vi "Header_Info_Str.vi"(8 "error in (no error)":errorcluster, 10 "Functions":i32, 11 "DefaultDev in":refnum<class "BaseDevice.lvclass">) -> (0 "error out":errorcluster, 1 "HdrInfoStr":string, 2 "InstrumentName":string, 3 "DefaultDev out":refnum<class "BaseDevice.lvclass">)   [LabVIEW 2019, in "BaseDevice.lvclass"]
uses:
  BaseDevice.lvclass
  BaseDevice.lvclass/BaseDevice.ctl
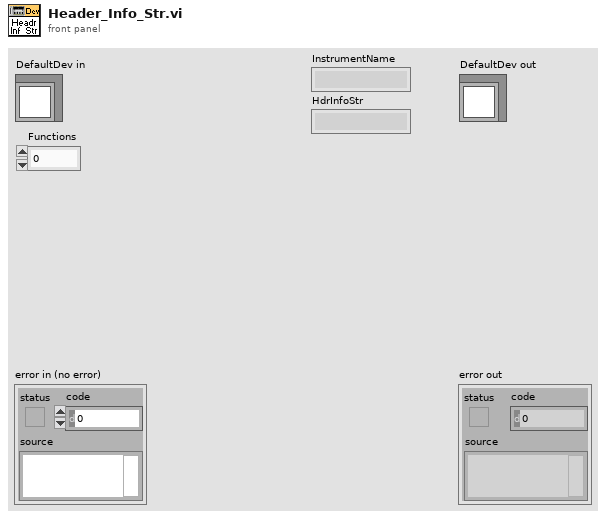
[diagram p1: front panel]
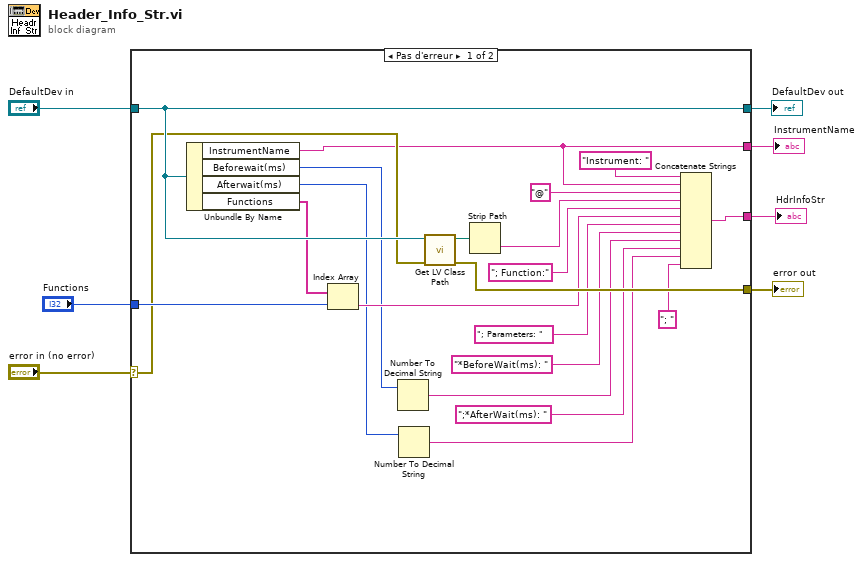
[diagram p0: block diagram]
diagram:
  n1 = case shown="Pas d'erreur" "error in (no error)" {
    selector: "error in (no error)" -> [w13 w30]
    tunnel: [w24 w30] -> w6
    tunnel: [w18 w29] -> w4
    tunnel: "DefaultDev in" -> [w18 w29]
    tunnel: [w12 _] -> w3
    tunnel: [w15 _] -> w2
    tunnel: "Functions" -> [w14 _]
    frame No Error {
      n2 = Unbundle By Name(w18) -> ("InstrumentName"=w12:string, "Beforewait(ms)"=w11:u32, "Afterwait(ms)"=w10:u32, "Functions"=w9:string[])
      n3 = Index Array(array=w9, index=w14) -> (element=w17:string)
      n4 = Number To Decimal String(number=w11) -> (decimal integer string=w22:string)  [unwired: 1 in]
      n5 = Number To Decimal String(number=w10) -> (decimal integer string=w20:string)  [unwired: 1 in]
      n6 = call <vilib>:"Get LV Class Path.vi"("error in (no error)"=w13, "object"=w18) -> ("error out"=w24:errorcluster, "class path"=w25:path)  [unwired: 8 in]
      n7 = Strip Path(path=w25) -> (name=w27:string)  [unwired: 1 out]
      n8 = Concatenate Strings("Instrument: " ("string"), w12, "@" ("string"), w27, "; Function:" ("Params"), w17, "; Parameters: " ("Params"), "*BeforeWait(ms): " ("Params"), w22, ";*AfterWait(ms): " ("Params"), w20, "; " ("chaîne")) -> (w15:string)
    }
    frame Error {
    }
  }
  "error out" <- w6
  "DefaultDev out" <- w4
  "InstrumentName" <- w3
  "HdrInfoStr" <- w2
